vi "CFTS-Read Connections.vi"(7 "Which":string="Analog Inputs", 11 "error in (no error)":errorcluster) -> (8 "endpoints":T1[](array[typedef]), 15 "error out":errorcluster)   [LabVIEW 2020]
uses:
  epl-vi-lib/Connection VIs/Typedefs/CM-Endpoint.ctl
  <vilib>/Utility/sysdir.llb/System Directory Type.ctl
  f00427ea-3526-4091-9261-4e0cbed7b5bb.vi
  <vilib>/Utility/config.llb/Read Key (I32).vi
  <vilib>/Comparison/Equal/Equal Functor/Equal Functor.lvclass
  <vilib>/Utility/config.llb/NI_LVConfig.lvlib
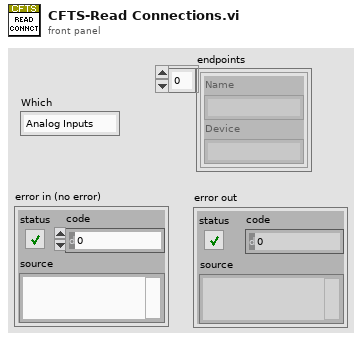
[diagram p1: front panel]
types:
  T1 = typedef "CM-Endpoint.ctl" = cluster{"Name":string, "Device":string}
  T2 = typedef "System Directory Type.ctl" = i32
  T3 = typedef "NI_LVConfig.lvlib/Config Data RefNum.ctl" = refnum<k1>
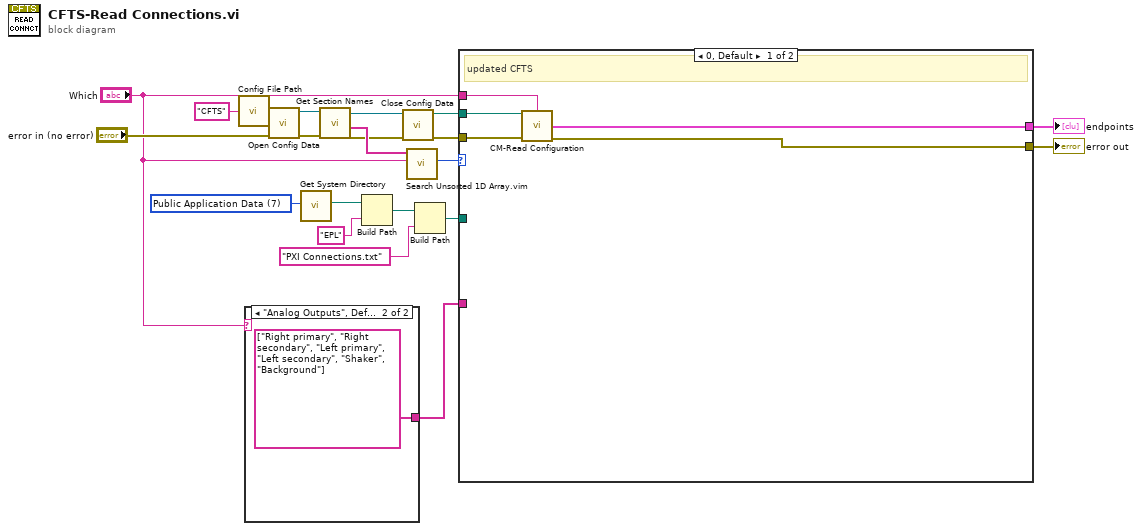
[diagram p0: block diagram]
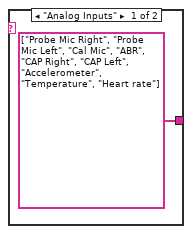
[diagram p2: hidden frame]
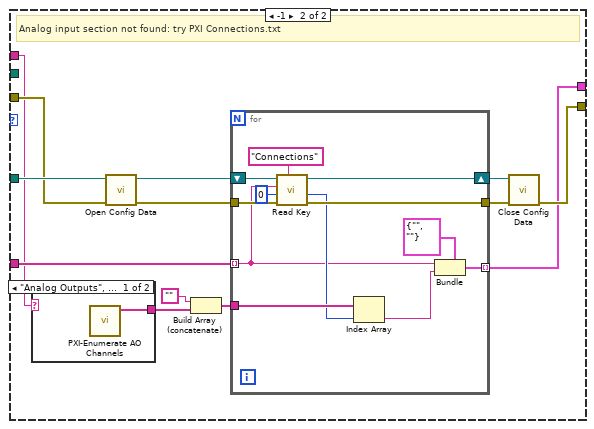
[diagram p3: hidden frame]
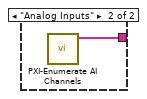
[diagram p4: hidden frame]
diagram:
  w9 = T2 7 items=["User Home", "User Desktop", "User Documents", "User Application Data", "User Preferences", "User Temporary", "Public Documents", "Public Application Data", "Public Preferences", "System Core Libraries", "System Installed Libraries", "Application Files", "Boot Volume Root"] ("system directory type")
  n1 = call "Config File Path.vi"("AppName"="CFTS") -> ("Default config file name"=w19:path)
  n2 = case shown="\"Analog Outputs\", Default" "Which" {
    tunnel: [string[] ["Probe Mic Right", "Probe Mic Left", "Cal Mic", "ABR", "CAP Right", "CAP Left", "Accelerometer", "Temperature", "Heart rate"] string[] ["Right primary", "Right secondary", "Left primary", "Left secondary", "Shaker", "Background"]] -> w21
    frame "Analog Inputs" {
    }
    frame "Analog Outputs", Default {
    }
  }
  n3 = call <vilib>:"Open Config Data.vi"("error in (no error)"="error in (no error)", "configuration file path"=w19) -> ("error out"=w17:errorcluster, "refnum"=w18:T3)  [unwired: 7 in, 1 out]
  n4 = call <vilib>:"Get System Directory.vi"("system directory type"=w9) -> ("system directory"=w8:path)  [unwired: 10 in]
  n5 = call <vilib>:"Get Section Names.vi"("error in (no error)"=w17, "refnum"=w18) -> ("error out"=w15:errorcluster, "section names"=w16:string[], "refnum out"=w14:T3)  [unwired: 7 in]
  n6 = Build Path(base path=w8, name or relative path="EPL") -> (appended path=w6:path)
  n7 = call <vilib>:"Close Config Data.vi"("error in (no error)"=w15, "refnum"=w14) -> ("error out"=w10:errorcluster, "file path"=w13:path)  [unwired: 8 in]
  n8 = call "Search Unsorted 1D Array.vim"("element"="Which", "unsorted 1D array"=w16) -> ("index of element"=w12:i32)  [unwired: 9 in]
  n9 = Build Path(base path=w6, name or relative path="PXI Connections.txt") -> (appended path=w4:path)
  n10 = case shown="0, Default" w12 {
    tunnel: w13 -> [w28 _]
    tunnel: w10 -> [w25 w38]
    tunnel: w4 -> [_ w39]
    tunnel: w21 -> [_ w35]
    tunnel: [w24 w32] -> w3
    tunnel: [w26 w30] -> w2
    tunnel: "Which" -> [w27 w29]
    frame 0, Default {
      # "updated CFTS"
      n11 = call "CM-Read Configuration.vi"("Connection File Path"=w28, "Section"=w27, "error in (no error)"=w25) -> ("Endpoints"=w26:T1[], "error out"=w24:errorcluster)  [unwired: 8 in, 3 out]
    }
    frame -1 {
      # "Analog input section not found: try PXI Connections.txt"
      n12 = case shown="\"Analog Outputs\", Default" w29 {
        tunnel: [w42 w43] -> w41
        frame "Analog Outputs", Default {
          n13 = call "PXI-Enumerate AO Channels.vi"() -> ("AO.PhysicalChans"=w42:tag[])  [unwired: 10 in, 1 out]
        }
        frame "Analog Inputs" {
          n14 = call "PXI-Enumerate AI Channels.vi"() -> ("AI.PhysicalChans"=w43:tag[])  [unwired: 10 in, 1 out]
        }
      }
      n15 = call <vilib>:"Open Config Data.vi"("error in (no error)"=w38, "configuration file path"=w39) -> ("error out"=w36:errorcluster, "refnum"=w37:T3)  [unwired: 7 in, 1 out]
      n16 = Build Array (concatenate)("", w41) -> (w31:string[])
      n17 = for {
        tunnel: w36 -> [w54]
        tunnel: w35 -> [w47] mode=indexing
        shift-right: [w51] -> w34
        shift-left: w37 -> [w55]
        tunnel: [w50] -> w33
        tunnel: w31 -> [w49]
        tunnel: [w45] -> w30 mode=indexing
        n18 = call-poly <vilib>:"Read Key.vi"("section"="Connections", "error in (no error)"=w54, "default value"=0, "key"=w47, "refnum"=w55) -> ("error out"=w50:errorcluster, "value"=w48:i32, "refnum out"=w51:T3)  [unwired: 3 in, 1 out]
        n19 = Index Array(array=w49, index=w48) -> (element=w46:string)
        n20 = Bundle(cluster=T1 {"Name"="", "Device"=""} ("Endpoint"), "Name"=w47, "Device"=w46) -> (w45:T1)
      }
      n21 = call <vilib>:"Close Config Data.vi"("error in (no error)"=w33, "refnum"=w34) -> ("error out"=w32:errorcluster)  [unwired: 8 in, 1 out]
    }
  }
  "error out" <- w3
  "endpoints" <- w2
